vi "GPS.vi"() -> ()   [LabVIEW 2020]
panel:
  out "Fecha":string
  out "Hora":string
  out "Ubicación":string
  out "A or V":string
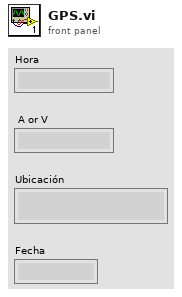
[diagram p1: front panel]
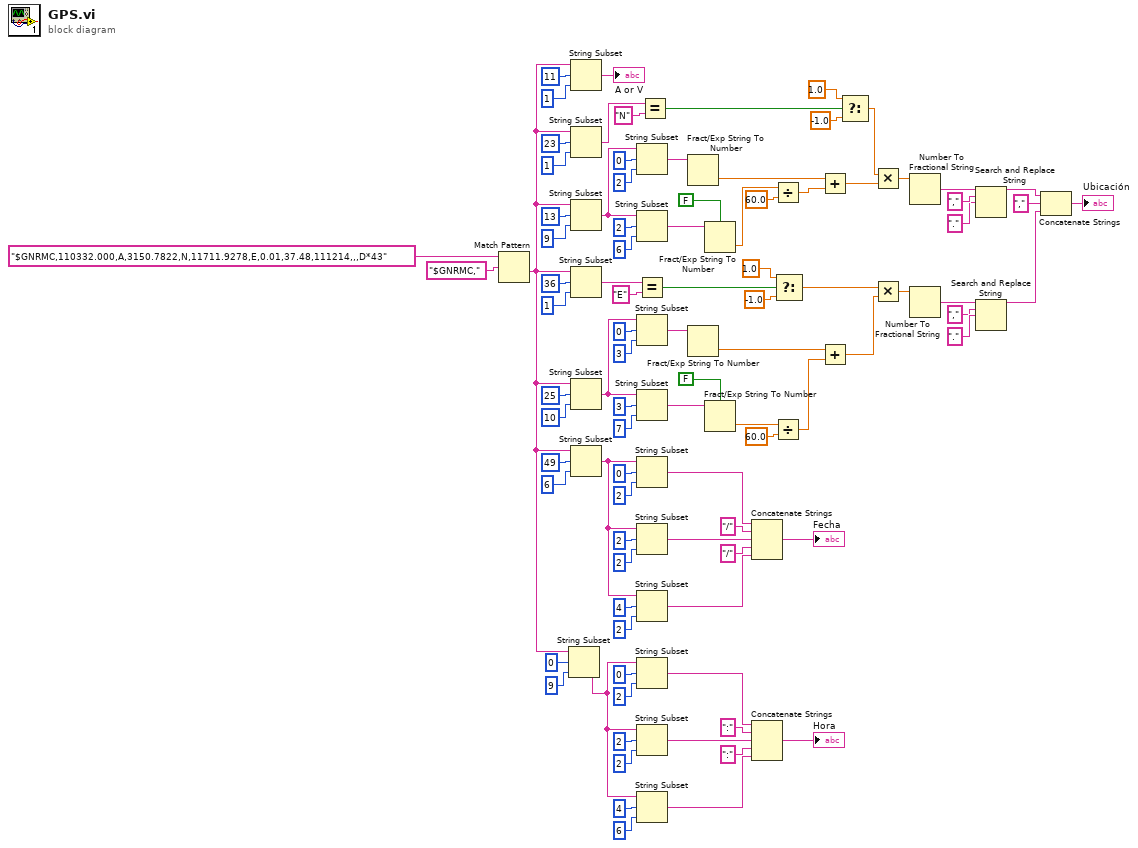
[diagram p0: block diagram]
diagram:
  n1 = Match Pattern(string="$GNRMC,110332.000,A,3150.7822,N,11711.9278,E,0.01,37.48,111214,,,D*43", regular expression="$GNRMC,") -> (after substring=w16:string)  [unwired: 1 in, 3 out]
  n2 = String Subset(string=w16, offset (0)=0, length (rest)=9 ("length (rest)")) -> (substring=w27:string)
  n3 = String Subset(string=w16, offset (0)=11, length (rest)=1 ("length (rest)")) -> (substring=→"A or V":string)
  n4 = String Subset(string=w16, offset (0)=23, length (rest)=1 ("length (rest)")) -> (substring=w72:string)
  n5 = String Subset(string=w16, offset (0)=13, length (rest)=9 ("length (rest)")) -> (substring=w84:string)
  n6 = String Subset(string=w16, offset (0)=36, length (rest)=1 ("length (rest)")) -> (substring=w46:string)
  n7 = String Subset(string=w16, offset (0)=25, length (rest)=10 ("length (rest)")) -> (substring=w56:string)
  n8 = String Subset(string=w16, offset (0)=49, length (rest)=6 ("length (rest)")) -> (substring=w9:string)
  n9 = String Subset(string=w84, offset (0)=0, length (rest)=2 ("length (rest)")) -> (substring=w80:string)
  n10 = String Subset(string=w84, offset (0)=2, length (rest)=6 ("length (rest)")) -> (substring=w81:string)
  n11 = Equal?(x=w46, y="E") -> (x = y?=w48:bool)
  n12 = String Subset(string=w56, offset (0)=0, length (rest)=3 ("length (rest)")) -> (substring=w60:string)
  n13 = String Subset(string=w56, offset (0)=3, length (rest)=7 ("length (rest)")) -> (substring=w59:string)
  n14 = String Subset(string=w9, offset (0)=0, length (rest)=2 ("length (rest)")) -> (substring=w6:string)
  n15 = String Subset(string=w9, offset (0)=2, length (rest)=2 ("length (rest)")) -> (substring=w4:string)
  n16 = String Subset(string=w9, offset (0)=4, length (rest)=2 ("length (rest)")) -> (substring=w2:string)
  n17 = String Subset(string=w27, offset (0)=0, length (rest)=2 ("length (rest)")) -> (substring=w24:string)
  n18 = String Subset(string=w27, offset (0)=2, length (rest)=2 ("length (rest)")) -> (substring=w22:string)
  n19 = String Subset(string=w27, offset (0)=4, length (rest)=6 ("length (rest)")) -> (substring=w20:string)
  n20 = Equal?(x=w72, y="N") -> (x = y?=w70:bool)
  n21 = Fract/Exp String To Number(string=w80) -> (number=w76:dbl)  [unwired: 3 in, 1 out]
  n22 = Fract/Exp String To Number(string=w60) -> (number=w64:dbl)  [unwired: 3 in, 1 out]
  n23 = Fract/Exp String To Number(use system decimal point (T)=FALSE, string=w81) -> (number=w78:dbl)  [unwired: 2 in, 1 out]
  n24 = Fract/Exp String To Number(use system decimal point (T)=FALSE, string=w59) -> (number=w62:dbl)  [unwired: 2 in, 1 out]
  n25 = Concatenate Strings(w6, "/" ("string"), w4, "/" ("string"), w2) -> (→"Fecha":string)
  n26 = Concatenate Strings(w24, ":" ("string"), w22, ":" ("string"), w20) -> (→"Hora":string)
  n27 = Divide(x=w78, y=60.0) -> (x/y=w75:dbl)
  n28 = Divide(x=w62, y=60.0) -> (x/y=w65:dbl)
  n29 = Select(t=1.0, s=w48, f=-1.0) -> (s? t:f=w51:dbl)
  n30 = Add(x=w76, y=w75) -> (x+y=w66:dbl)
  n31 = Add(x=w64, y=w65) -> (x+y=w45:dbl)
  n32 = Select(t=1.0, s=w70, f=-1.0) -> (s? t:f=w67:dbl)
  n33 = Multiply(x=w67, y=w66) -> (x*y=w42:dbl)
  n34 = Multiply(x=w51, y=w45) -> (x*y=w41:dbl)
  n35 = Number To Fractional String(number=w42) -> (F-format string=w40:string)  [unwired: 3 in]
  n36 = Number To Fractional String(number=w41) -> (F-format string=w35:string)  [unwired: 3 in]
  n37 = Search and Replace String(input string=w40, search string=",", replace string="." ("replace string (\"\")")) -> (result string=w32:string)  [unwired: 5 in, 3 out]
  n38 = Search and Replace String(input string=w35, search string=",", replace string="." ("replace string (\"\")")) -> (result string=w34:string)  [unwired: 5 in, 3 out]
  n39 = Concatenate Strings(w32, "," ("string"), w34) -> (→"Ubicación":string)
